vi "daqio.vi"   [LabVIEW 2013, in "daqio minimal.lvlib"]
uses:
  daqio minimal.lvlib
panel:
  # "opening the Quick Reference Guide..."
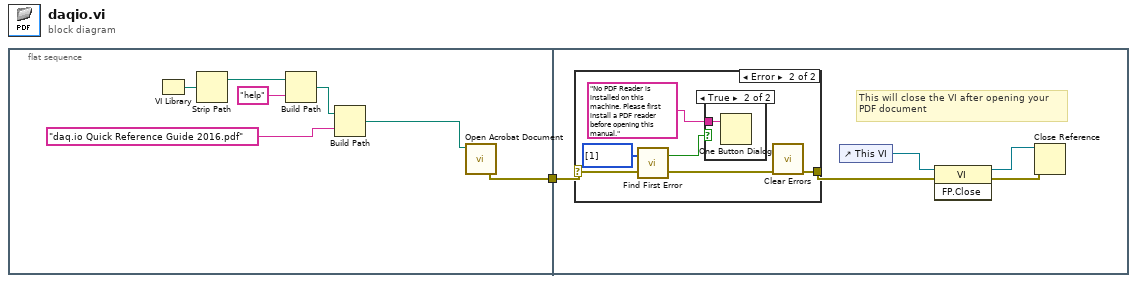
[diagram p0: block diagram]
diagram:
  n1 = flat-sequence {
    tunnel: [w8] -> w1
    tunnel: w1 -> [w10]
    frame #0 {
      n2 = VI Library() -> (path=w7:path)
      n3 = Strip Path(path=w7) -> (stripped path=w6:path)  [unwired: 1 out]
      n4 = Build Path(base path=w6, name or relative path="help") -> (appended path=w4:path)
      n5 = Build Path(base path=w4, name or relative path="daq.io Quick Reference Guide 2016.pdf") -> (appended path=w2:path)
      n6 = call <vilib>:"Open Acrobat Document.vi"("acrobat document"=w2) -> ("error out"=w8:errorcluster)  [unwired: 6 in]
    }
    frame #1 {
      # "This will close the VI after opening your\nPDF document"
      n7 = case shown="Error" w10 {
        selector: w10 -> [w14 w20]
        tunnel: [w14 w17] -> w9
        frame No Error {
        }
        frame Error {
          n8 = call <vilib>:"Find First Error.vi"("error in (no error)"=w20, "error codes"=i32[] [1]) -> ("error out"=w18:errorcluster, "error?"=w16:bool)  [unwired: 2 in]
          n9 = case shown="True" w16 {
            tunnel: "No PDF Reader is installed on this machine. Please first install a PDF reader before opening this manual." -> [_ w21]
            frame False {
            }
            frame True {
              n10 = One Button Dialog(message=w21) -> ()  [unwired: 1 in, 1 out]
            }
          }
          n11 = call <vilib>:"Clear Errors.vi"("error in (no error)"=w18) -> ("error out"=w17:errorcluster)  [unwired: 6 in]
        }
      }
      n12 = control-ref of="This VI"() -> (w11:refnum<vi>)
      n13 = invoke class="VI" method="FP.Close"(reference=w11, error in=w9) -> (reference out=w13:refnum<vi>, error out=w12:errorcluster)  [unwired: 1 in, 1 out]
      n14 = Close Reference(reference=w13, error in (no error)=w12) -> ()  [unwired: 1 out]
    }
  }
